vi "MotorMain.vi"() -> ()   [LabVIEW 2011]
uses:
  Modules/PIMotorController/PI_Axis_list.ctl
  Modules/PIMotorController/PI_Axis.ctl
  Main/Motors/MotorConfigType.ctl
  Main/Motors/MotorPosType.ctl
  Main/Typedefs/XYf.ctl
  Main/Motors/MotorPosFlagsType.ctl
panel:
  out "Conn. \nAxes 2":string[](array[string])
  out "Conn. Axes":string[](array[string])
  out "All conn. axes":string[](array[string])
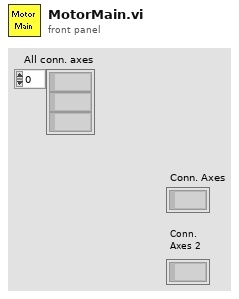
[diagram p1: front panel]
types:
  T1 = typedef "PI_Axis_list.ctl" = cluster{"Piezo X":T2, "Piezo Y":T2, "Piezo Z":T2, "Magnet Z":T2, "Magnet Rotation":T2, "Objective X":T2, "Objective Y":T2}
  T2 = typedef "PI_Axis.ctl" = cluster{"System #":i32, "Axis ID":string, "Multiplier":dbl}
  T3 = typedef "MotorConfigType.ctl" = cluster{"Offset":T4, "Maximum pos":T4, "Min limited?":T6, "Max limited?":T6, "Has velocity support":T6, "Default velocity":T4}
  T4 = typedef "MotorPosType.ctl" = cluster{"Magnet Z":dbl, "Magnet rotation":dbl, "Camera":T5, "Piezo XY":T5, "Piezo Z":dbl, "Coil XY":T5}
  T5 = typedef "XYf.ctl" = cluster{"X":sgl, "Y":sgl}
  T6 = typedef "MotorPosFlagsType.ctl" = cluster{"Magnet Z":bool, "Magnet rotation":bool, "Camera":cluster{"X":bool, "Y":bool}, "Piezo XY":cluster{"X":bool, "Y":bool}, "Piezo Z":bool, "Coil XY":cluster{"X":bool, "Y":bool}}
  T7 = typedef "GCS_Interface.ctl" = cluster{"MOV":refnum<vi>, "VEL":refnum<vi>, "VEL?":refnum<vi>, "POS?":refnum<vi>, "TMX?":refnum<vi>, "#7 (Ready?)":refnum<vi>, "FPL":refnum<vi>, "FNL":refnum<vi>}
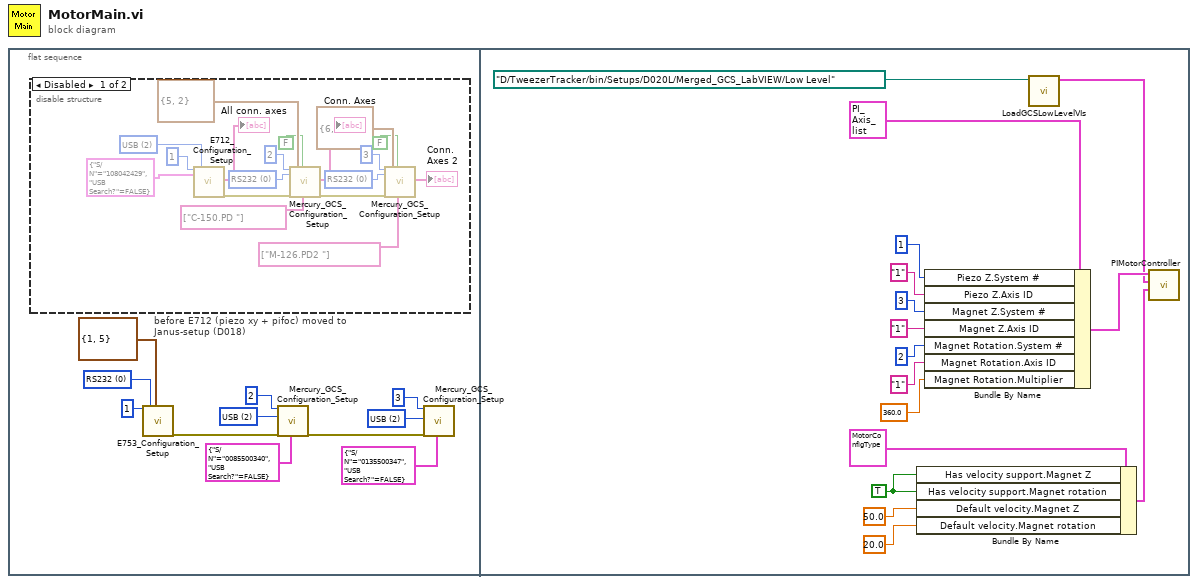
[diagram p0: block diagram]
diagram:
  n1 = flat-sequence {
    frame #0 {
      w2 = u16 2 items=["RS232", "RS232 DaisyChain", "USB", "USB_DaisyChain"] ("Interface")
      w6 = u16 2 items=["RS232", "RS232 DaisyChain", "USB", "USB_DaisyChain"] ("Interface")
      w10 = u16 0 items=["RS232", "TCP/IP"] ("Interface")
      n2 = disable-structure "before E712 (piezo xy + pifoc) moved to Janus-setup (D018)" shown="Disabled" {
        frame Disabled {
          w22 = u16 0 items=["RS232", "RS232 DaisyChain", "USB", "USB_DaisyChain"] ("Interface")
          w24 = u16 0 items=["RS232", "RS232 DaisyChain", "USB", "USB_DaisyChain"] ("Interface")
          w28 = u16 2 items=["RS232", "TCP/IP", "USB"] ("Interface")
          n3 = call "E712_Configuration_Setup.vi"("System no."=1, "USB settings"=cluster{"S/N":string, "USB Search?":bool} {"S/N"="108042429", "USB Search?"=FALSE}, "Interface"=w28) -> ("All conn. axes"=→"All conn. axes":string[], "error out"=w25:errorcluster)  [unwired: 12 in, 3 out]
          n4 = call "Mercury_GCS_Configuration_Setup.vi"("System no."=2, "error in"=w25, "RS232 settings"=cluster{"Portnumber":i32, "Baudrate":i32} {"Portnumber"=5, "Baudrate"=2}, "DaisyChain settings"=FALSE ("Use dialog to define\nconnected stages?"), "USB settings"=string[] ["C-150.PD "] ("Stage names input"), "Reference Move"=w24) -> ("Conn. \nAxes"=→"Conn. Axes":string[], "error out"=w19:errorcluster)  [unwired: 7 in, 5 out]
          n5 = call "Mercury_GCS_Configuration_Setup.vi"("System no."=3, "error in"=w19, "RS232 settings"=cluster{"Portnumber":i32, "Baudrate":i32} {"Portnumber"=6, "Baudrate"=2}, "DaisyChain settings"=FALSE ("Use dialog to define\nconnected stages?"), "USB settings"=string[] ["M-126.PD2 "] ("Stage names input"), "Reference Move"=w22) -> ("Conn. \nAxes"=→"Conn. \nAxes 2":string[])  [unwired: 7 in, 6 out]
        }
        frame Enabled {
        }
      }
      n6 = call "E753_Configuration_Setup.vi"("System no."=1, "Interface"=w10, "RS232 settings"=cluster{"Portnumber":i32, "Baudrate":u16} {"Portnumber"=1, "Baudrate"=5}) -> ("error out"=w8:errorcluster)  [unwired: 11 in, 5 out]
      n7 = call "Mercury_GCS_Configuration_Setup.vi"("System no."=2, "Interface"=w6, "error in"=w8, "USB settings"=cluster{"S/N":string, "USB Search?":bool} {"S/N"="0085500340", "USB Search?"=FALSE}) -> ("error out"=w4:errorcluster)  [unwired: 9 in, 6 out]
      n8 = call "Mercury_GCS_Configuration_Setup.vi"("System no."=3, "Interface"=w2, "error in"=w4, "USB settings"=cluster{"S/N":string, "USB Search?":bool} {"S/N"="0135500347", "USB Search?"=FALSE}) -> ()  [unwired: 9 in, 7 out]
    }
    frame #1 {
      w41 = TRUE ("Has velocity support.Magnet Z")
      n9 = Bundle By Name(cluster=T3 {"Offset"={"Magnet Z"=0.0, "Magnet rotation"=0.0, "Camera"={"X"=0.0, "Y"=0.0}, "Piezo XY"={"X"=0.0, "Y"=0.0}, "Piezo Z"=0.0, "Coil XY"={"X"=0.0, "Y"=0.0}}, "Maximum pos"={"Magnet Z"=0.0, "Magnet rotation"=0.0, "Camera"={"X"=0.0, "Y"=0.0}, "Piezo XY"={"X"=0.0, "Y"=0.0}, "Piezo Z"=0.0, "Coil XY"={"X"=0.0, "Y"=0.0}}, "Min limited?"={"Magnet Z"=FALSE, "Magnet rotation"=FALSE, "Camera"={"X"=FALSE, "Y"=FALSE}, "Piezo XY"={"X"=FALSE, "Y"=FALSE}, "Piezo Z"=FALSE, "Coil XY"={"X"=FALSE, "Y"=FALSE}}, "Max limited?"={"Magnet Z"=FALSE, "Magnet rotation"=FALSE, "Camera"={"X"=FALSE, "Y"=FALSE}, "Piezo XY"={"X"=FALSE, "Y"=FALSE}, "Piezo Z"=FALSE, "Coil XY"={"X"=FALSE, "Y"=FALSE}}, "Has velocity support"={"Magnet Z"=TRUE, "Magnet rotation"=TRUE, "Camera"={"X"=FALSE, "Y"=FALSE}, "Piezo XY"={"X"=FALSE, "Y"=FALSE}, "Piezo Z"=FALSE, "Coil XY"={"X"=FALSE, "Y"=FALSE}}, "Default velocity"={"Magnet Z"=0.0, "Magnet rotation"=0.0, "Camera"={"X"=0.0, "Y"=0.0}, "Piezo XY"={"X"=0.0, "Y"=0.0}, "Piezo Z"=0.0, "Coil XY"={"X"=0.0, "Y"=0.0}}} ("MotorConfig"), "Has velocity support.Magnet Z"=w41, "Has velocity support.Magnet rotation"=w41, "Default velocity.Magnet Z"=50.0, "Default velocity.Magnet rotation"=20.0) -> (w30:T3)
      n10 = Bundle By Name(cluster=T1 {"Piezo X"={"System #"=0, "Axis ID"="", "Multiplier"=1.0}, "Piezo Y"={"System #"=0, "Axis ID"="", "Multiplier"=1.0}, "Piezo Z"={"System #"=0, "Axis ID"="", "Multiplier"=1.0}, "Magnet Z"={"System #"=0, "Axis ID"="", "Multiplier"=1.0}, "Magnet Rotation"={"System #"=0, "Axis ID"="", "Multiplier"=1.0}, "Objective X"={"System #"=0, "Axis ID"="", "Multiplier"=1.0}, "Objective Y"={"System #"=0, "Axis ID"="", "Multiplier"=1.0}} ("PI Axis config"), "Piezo Z.System #"=1, "Piezo Z.Axis ID"="1", "Magnet Z.System #"=3, "Magnet Z.Axis ID"="1", "Magnet Rotation.System #"=2, "Magnet Rotation.Axis ID"="1", "Magnet Rotation.Multiplier"=360.0) -> (w32:T1)
      n11 = call "LoadGCSLowLevelVIs.vi"("GCS Merged Drivers Low-Level Path"=path "D:/TweezerTracker/bin/Setups/D020L/Merged_GCS_LabVIEW/Low Level") -> ("PI GCS Function\nReferences"=w31:T7)  [unwired: 10 in]
      n12 = call "PIMotorController.vi"("MotorConfig"=w30, "PI GCS Function\nReferences"=w31, "PI Axis config"=w32) -> ()  [unwired: 9 in]
    }
  }
